vi "To Integer Tree Data.vi"(10 "Integer":i64) -> (3 "Integer Tree Data":refnum<class "Int.lvclass">)   [LabVIEW 2017, in "Tree API.lvlib" / "Int.lvclass"]
doc: "Convert an Integer value to Tree Data type."
uses:
  Int.lvclass
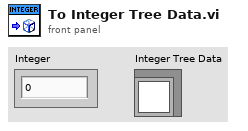
[diagram p1: front panel]
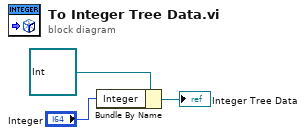
[diagram p0: block diagram]
diagram:
  n1 = Bundle By Name(cluster=refnum<class "Int.lvclass"> refnum ("Int in"), "Integer"="Integer") -> (→"Integer Tree Data":refnum<class "Int.lvclass">)
